vi "Periodicity.vi"() -> ()   [LabVIEW 2014]
panel:
  out "mag of X(w+2*pi*k)":cluster{"-pi to pi":dbl[], "Magnitude op":dbl[]}(graph)
  out "mag of X(w)":cluster{"-pi to pi":dbl[], "Magnitude op":dbl[]}(graph)
  in  "Boolean":bool
  out "X(w+2pi*k)":cluster{"-pi to pi":dbl[], dbl[]}(graph)
  out "X(w)":cluster{"-pi to pi":dbl[], "Magnitude op":dbl[]}(graph)
  in  "k":dbl
  out "mag{X(w)}":dbl[](array[numeric])
  out "X(w)":cdb[](array[numeric])
  out "X(w+2pi*k)":cdb[](array[numeric])
  in  "x(n)":dbl[](array[numeric])
  out "mag{X(w+2pi*k)}":dbl[](array[numeric])
  # "Instructions"
  # "if \nDTFT{x(n)} ----> X(w)\nthen\nX(w+2*pi*k) = X(w)"
  # "1. enter the array values as input sequence\n2. enter the value of k\n3. verify the output from the graph accoding to the property\n4. change the value of k to decimal number to see the deviation"
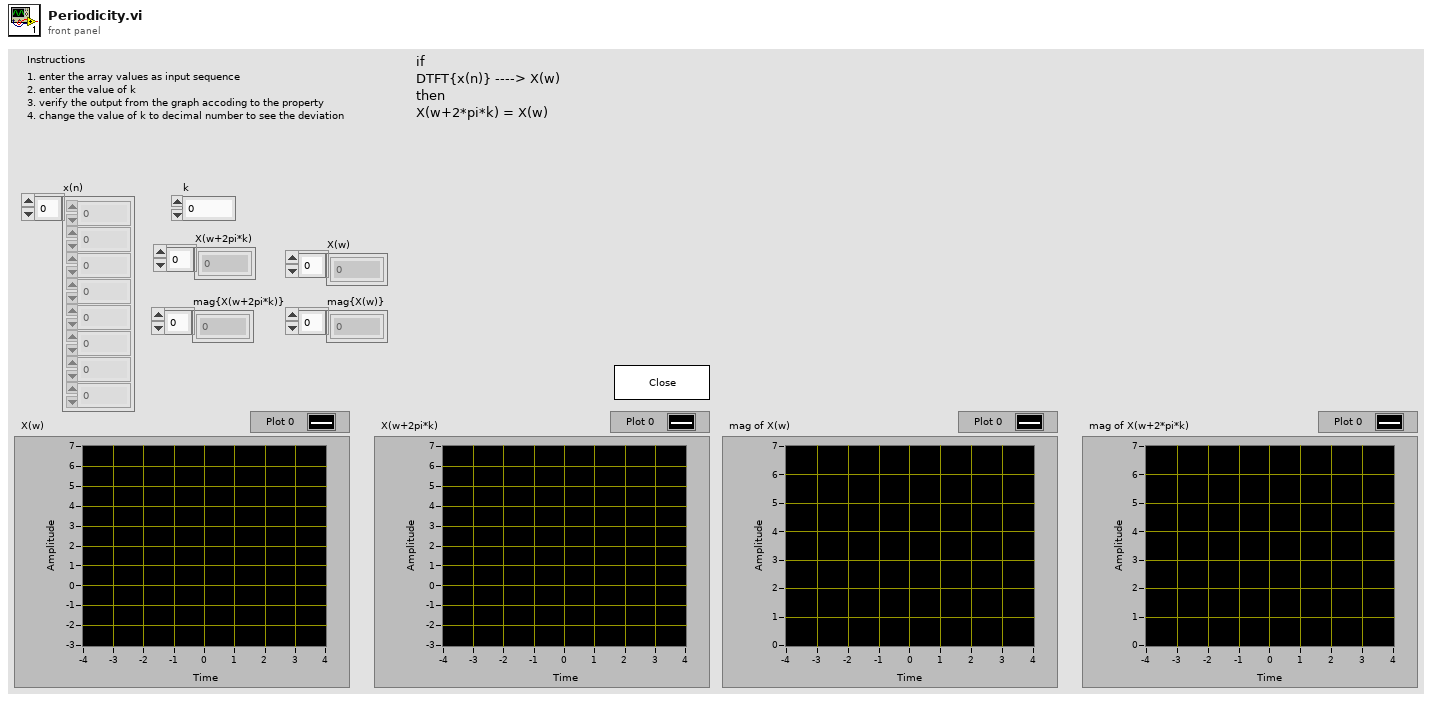
[diagram p1: front panel]
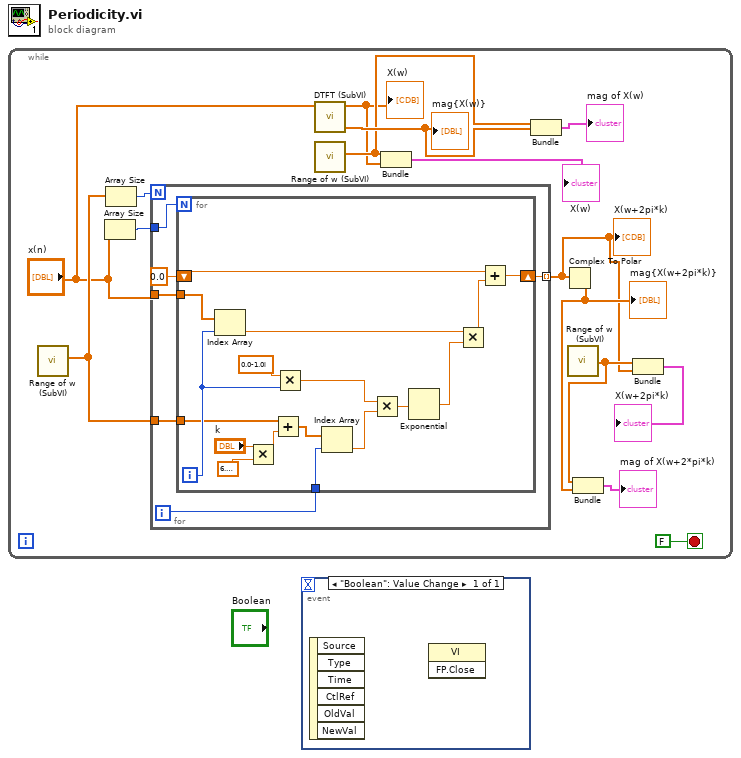
[diagram p0: block diagram]
diagram:
  n1 = while {
    stop <- FALSE stop-if-true
    n2 = call "Range of w (SubVI).vi"() -> ("-pi to pi"=w14:dbl[])  [unwired: 11 in]
    n3 = Array Size(array="x(n)") -> (size(s)=w15:i32)
    n4 = Array Size(array=w14) -> (size(s)=w13:i32)
    n5 = for {
      N: w13 -> [_]
      tunnel: w14 -> [w20]
      tunnel: w15 -> [w19]
      tunnel: "x(n)" -> [w17]
      tunnel: [w16] -> w2 mode=indexing
      i -> [w21]
      n6 = for {
        N: w19 -> [_]
        tunnel: w21 -> [w37]
        tunnel: w20 -> [w26]
        shift-right: [w31] -> w16
        shift-left: 0.0 -> [w30]
        tunnel: w17 -> [w27]
        i -> [w28]
        n7 = Index Array(array=w27, index=w28) -> (element=w29:dbl)
        n8 = Multiply(x="k", y=6.283185307179586) -> (x*y=w23:dbl)
        n9 = Add(x=w26, y=w23) -> (x+y=w25:dbl[])
        n10 = Multiply(x=cdb 0.0-1.0i, y=w28) -> (x*y=w36:cdb)
        n11 = Index Array(array=w25, index=w37) -> (element=w35:dbl)
        n12 = Multiply(x=w36, y=w35) -> (x*y=w34:cdb)
        n13 = Exponential(1:w34) -> (0:w33:cdb)
        n14 = Multiply(x=w29, y=w33) -> (x*y=w32:cdb)
        n15 = Add(x=w30, y=w32) -> (x+y=w31:cdb)
      }
    }
    "X(w+2pi*k)" <- w2
    n16 = call "DTFT (SubVI).vi"("ip array"="x(n)") -> ("Magnitude op"=w8:dbl[], "DTFT op"=w1:cdb[])  [unwired: 9 in]
    "X(w)" <- w1
    "mag{X(w)}" <- w8
    n17 = call "Range of w (SubVI).vi"() -> ("-pi to pi"=w7:dbl[])  [unwired: 11 in]
    n18 = Bundle("-pi to pi"=w7, "DTFT op"=w1) -> (→"X(w)":cluster{"-pi to pi":dbl[], "DTFT op":cdb[]})  [unwired: 1 in]
    n19 = Bundle("-pi to pi"=w7, "Magnitude op"=w8) -> (→"mag of X(w)":cluster{"-pi to pi":dbl[], "Magnitude op":dbl[]})  [unwired: 1 in]
    n20 = Complex To Polar(r * e^(i*theta)=w2) -> (r=w3:dbl[])  [unwired: 1 out]
    "mag{X(w+2pi*k)}" <- w3
    n21 = call "Range of w (SubVI).vi"() -> ("-pi to pi"=w4:dbl[])  [unwired: 11 in]
    n22 = Bundle("-pi to pi"=w4, w3) -> (→"mag of X(w+2*pi*k)":cluster{"-pi to pi":dbl[], dbl[]})  [unwired: 1 in]
    n23 = Bundle("-pi to pi"=w4, w2) -> (→"X(w+2pi*k)":cluster{"-pi to pi":dbl[], cdb[]})  [unwired: 1 in]
  }
  n24 = event shown="[0] \"Boolean\": Value Change" {
    selector: _ -> [_]
    dyn-events: _ -> [_]
    timeout: _ -> [_]
    event "Boolean": Value Change {
      n25 = event-data() -> ()  [unwired: 1 in, 6 out]
      n26 = invoke class="VI" method="FP.Close"() -> ()  [unwired: 3 in, 3 out]
    }
  }
